vi "map_XY_proc_marmo.vi"() -> ()   [LabVIEW 2011]
panel:
  in  "go to z meas":bool
  in  "find z pos 3":bool
  in  "find z pos 2":bool
  in  "find z pos":bool
  in  "find y pos":bool
  in  "find x pos":bool
  in  "zero y":bool
  in  "zero x":bool
  in  "zero Z":bool
  in  "stop":bool
  out "command":string
  out "output":string
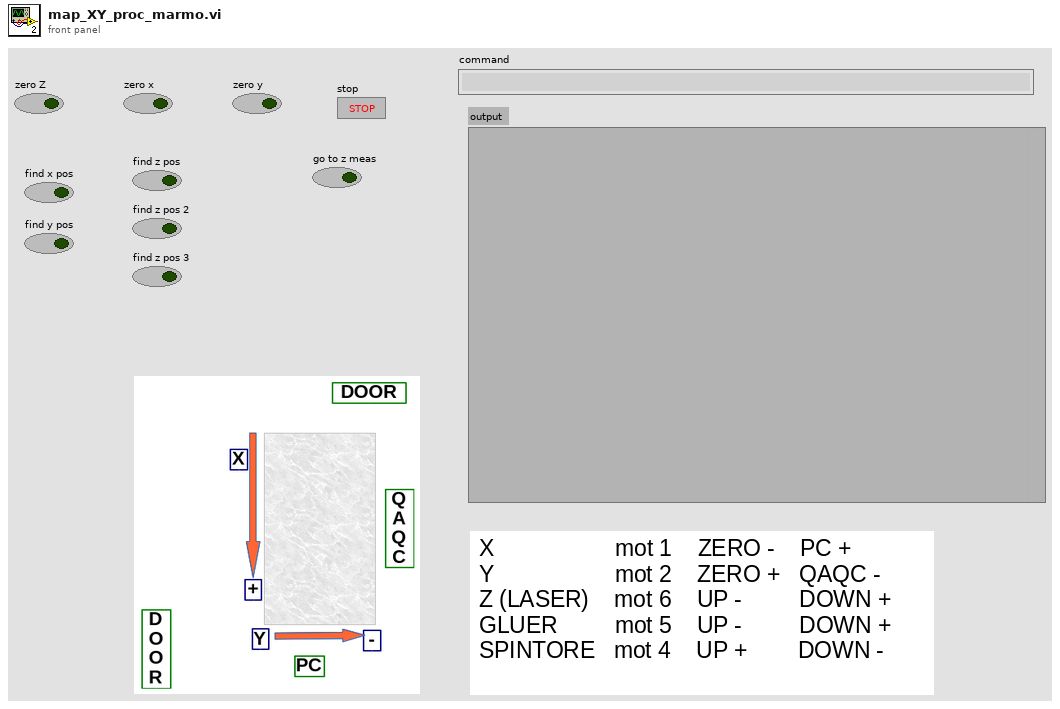
[diagram p1: front panel]
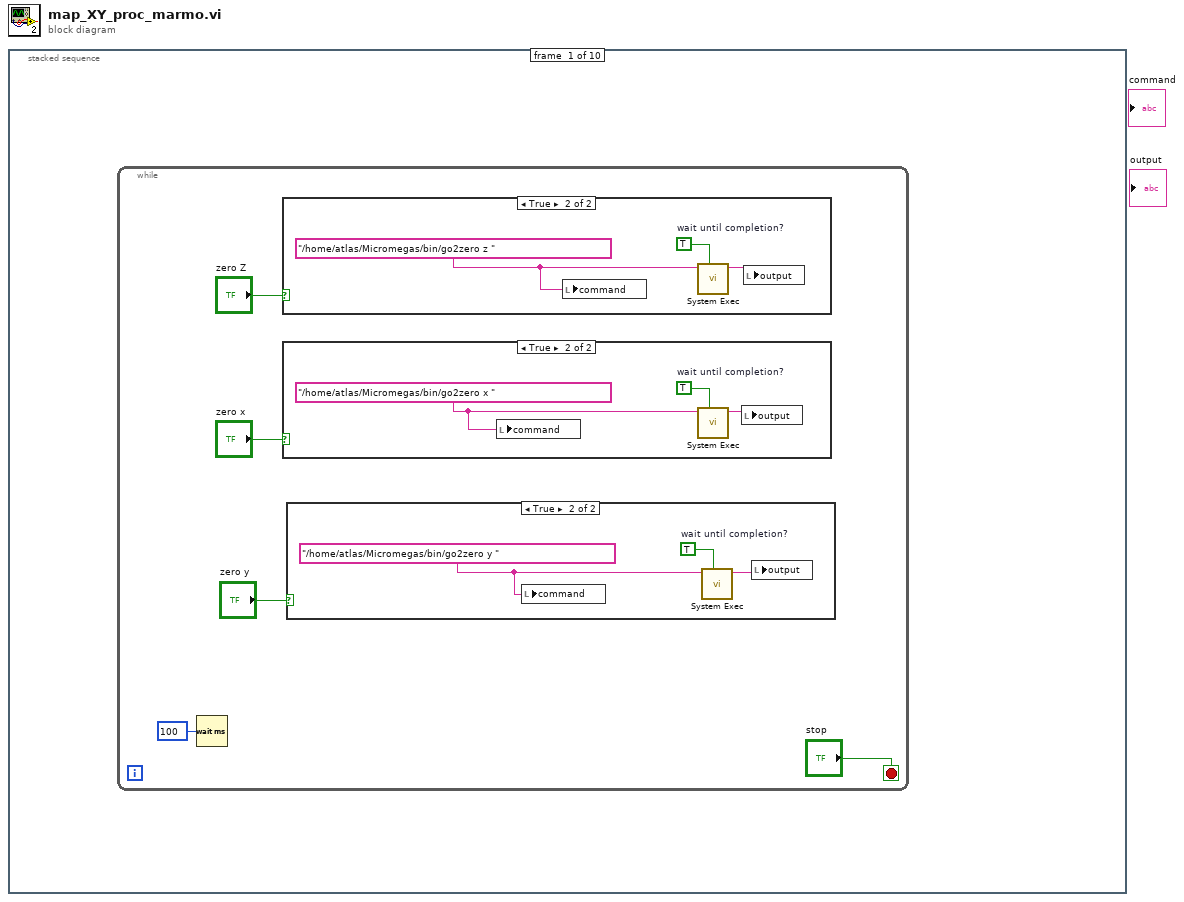
[diagram p0: block diagram]
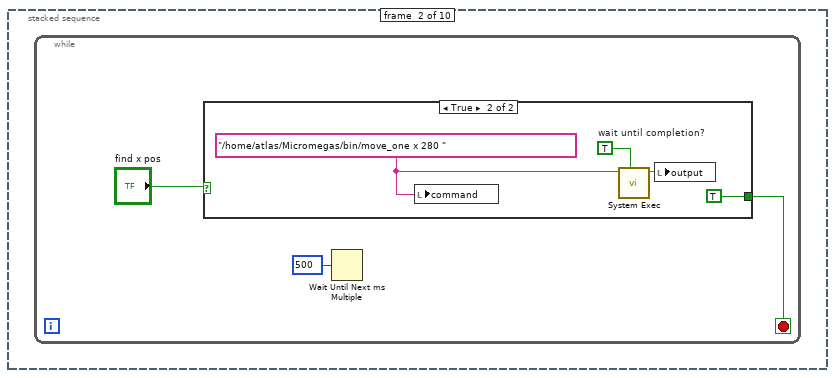
[diagram p5: hidden frame]
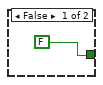
[diagram p6: hidden frame]
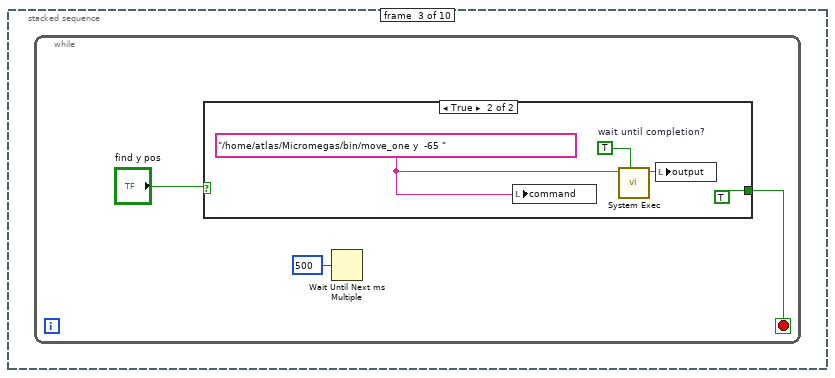
[diagram p7: hidden frame]
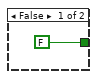
[diagram p8: hidden frame]
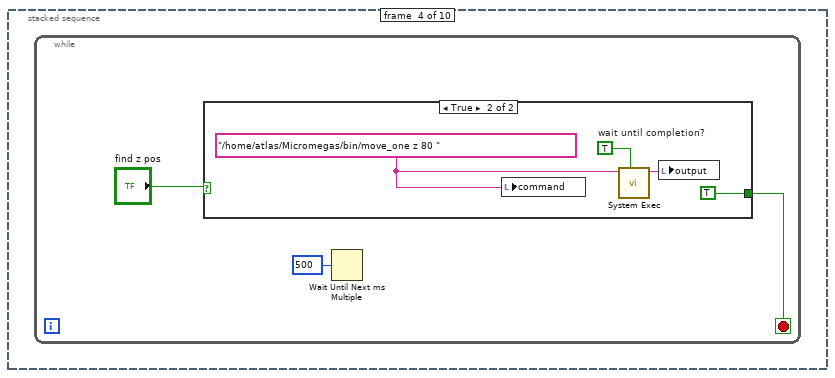
[diagram p9: hidden frame]
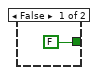
[diagram p10: hidden frame]
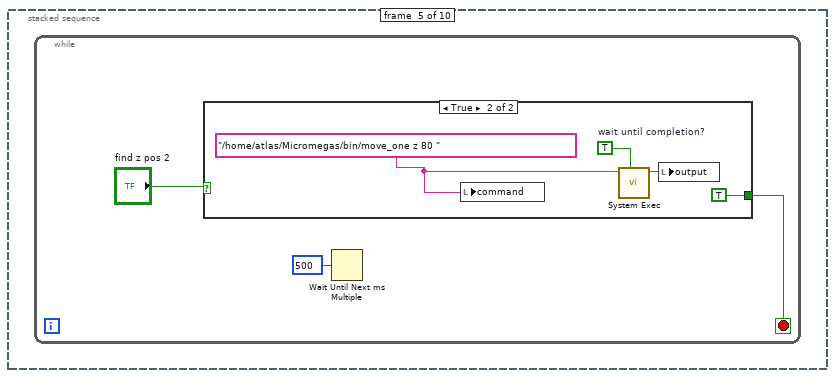
[diagram p11: hidden frame]
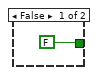
[diagram p12: hidden frame]
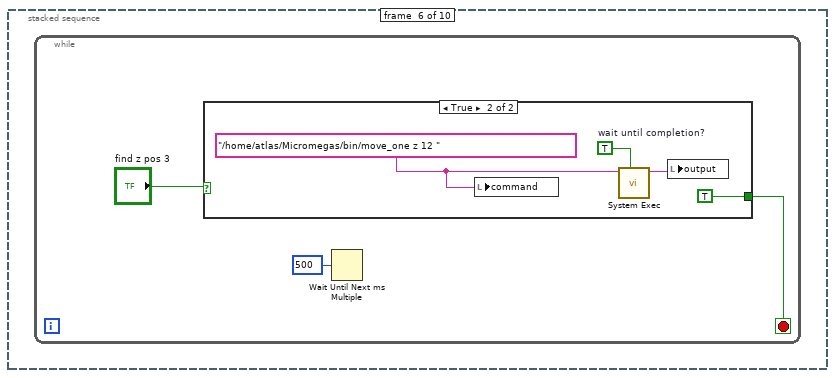
[diagram p13: hidden frame]
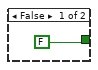
[diagram p14: hidden frame]
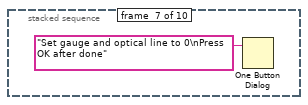
[diagram p15: hidden frame]
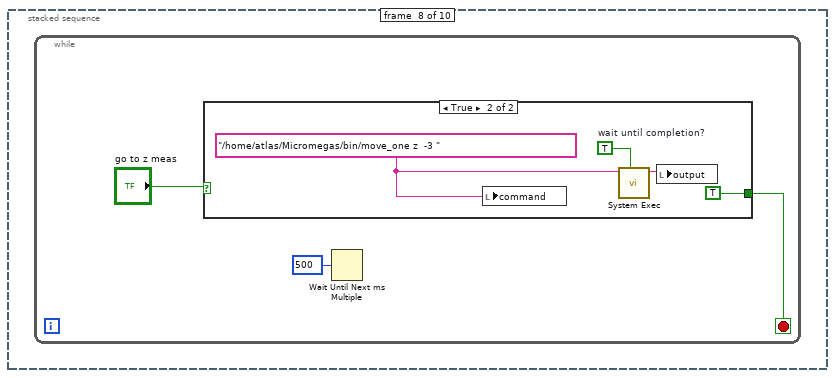
[diagram p16: hidden frame]
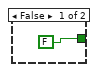
[diagram p17: hidden frame]
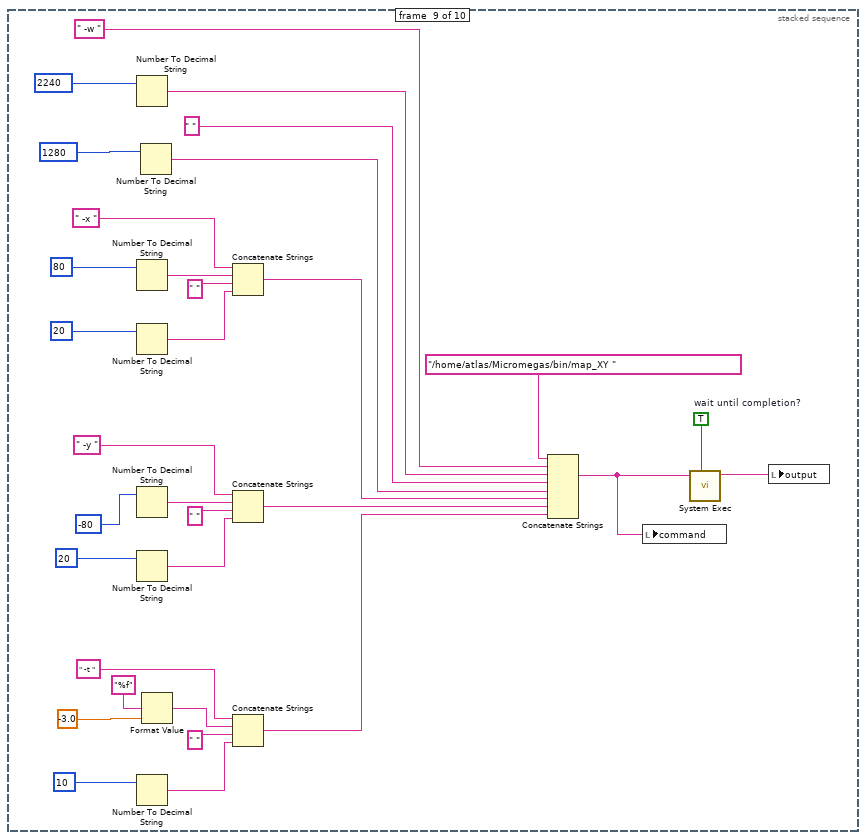
[diagram p18: hidden frame]
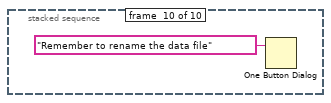
[diagram p19: hidden frame]
diagram:
  n1 = stacked-sequence {
    frame #0 {
      n2 = while {
        stop <- "stop" stop-if-true
        n3 = Wait (ms)(milliseconds to wait=u32 100) -> ()  [unwired: 1 out]
        n4 = case shown="True" "zero Z" {
          frame False {
          }
          frame True {
            w13 = "/home/atlas/Micromegas/bin/go2zero z " ("string")
            w14 = TRUE  # wait until completion?
            n5 = local write "command"(w13) -> ()
            n6 = call <vilib>:"System Exec.vi"("wait until completion? (T)"=w14, "command line"=w13) -> ("standard output"=w12:string)  [unwired: 6 in, 3 out]
            n7 = local write "output"(w12) -> ()
          }
        }
        n8 = case shown="True" "zero x" {
          frame False {
          }
          frame True {
            w10 = "/home/atlas/Micromegas/bin/go2zero x " ("string")
            w11 = TRUE  # wait until completion?
            n9 = local write "command"(w10) -> ()
            n10 = call <vilib>:"System Exec.vi"("wait until completion? (T)"=w11, "command line"=w10) -> ("standard output"=w9:string)  [unwired: 6 in, 3 out]
            n11 = local write "output"(w9) -> ()
          }
        }
        n12 = case shown="True" "zero y" {
          frame False {
          }
          frame True {
            w7 = "/home/atlas/Micromegas/bin/go2zero y " ("string")
            w8 = TRUE  # wait until completion?
            n13 = local write "command"(w7) -> ()
            n14 = call <vilib>:"System Exec.vi"("wait until completion? (T)"=w8, "command line"=w7) -> ("standard output"=w6:string)  [unwired: 6 in, 3 out]
            n15 = local write "output"(w6) -> ()
          }
        }
      }
    }
    frame #1 {
      n16 = while {
        stop <- w15 stop-if-true
        n17 = case shown="True" "find x pos" {
          tunnel: [FALSE TRUE] -> w15
          frame False {
          }
          frame True {
            w20 = "/home/atlas/Micromegas/bin/move_one x 280 " ("string")
            w22 = TRUE  # wait until completion?
            n18 = local write "command"(w20) -> ()
            n19 = call <vilib>:"System Exec.vi"("wait until completion? (T)"=w22, "command line"=w20) -> ("standard output"=w21:string)  [unwired: 6 in, 3 out]
            n20 = local write "output"(w21) -> ()
          }
        }
        n21 = Wait Until Next ms Multiple(millisecond multiple=u32 500) -> ()  [unwired: 1 out]
      }
    }
    frame #2 {
      n22 = while {
        stop <- w23 stop-if-true
        n23 = case shown="True" "find y pos" {
          tunnel: [FALSE TRUE] -> w23
          frame False {
          }
          frame True {
            w28 = "/home/atlas/Micromegas/bin/move_one y  -65 " ("string")
            w30 = TRUE  # wait until completion?
            n24 = local write "command"(w28) -> ()
            n25 = call <vilib>:"System Exec.vi"("wait until completion? (T)"=w30, "command line"=w28) -> ("standard output"=w29:string)  [unwired: 6 in, 3 out]
            n26 = local write "output"(w29) -> ()
          }
        }
        n27 = Wait Until Next ms Multiple(millisecond multiple=u32 500) -> ()  [unwired: 1 out]
      }
    }
    frame #3 {
      n28 = while {
        stop <- w31 stop-if-true
        n29 = case shown="True" "find z pos" {
          tunnel: [FALSE TRUE] -> w31
          frame False {
          }
          frame True {
            w36 = "/home/atlas/Micromegas/bin/move_one z 80 " ("string")
            w38 = TRUE  # wait until completion?
            n30 = local write "command"(w36) -> ()
            n31 = call <vilib>:"System Exec.vi"("wait until completion? (T)"=w38, "command line"=w36) -> ("standard output"=w37:string)  [unwired: 6 in, 3 out]
            n32 = local write "output"(w37) -> ()
          }
        }
        n33 = Wait Until Next ms Multiple(millisecond multiple=u32 500) -> ()  [unwired: 1 out]
      }
    }
    frame #4 {
      n34 = while {
        stop <- w39 stop-if-true
        n35 = case shown="True" "find z pos 2" {
          tunnel: [FALSE TRUE] -> w39
          frame False {
          }
          frame True {
            w45 = "/home/atlas/Micromegas/bin/move_one z 80 " ("string")
            w46 = TRUE  # wait until completion?
            n36 = local write "command"(w45) -> ()
            n37 = call <vilib>:"System Exec.vi"("wait until completion? (T)"=w46, "command line"=w45) -> ("standard output"=w44:string)  [unwired: 6 in, 3 out]
            n38 = local write "output"(w44) -> ()
          }
        }
        n39 = Wait Until Next ms Multiple(millisecond multiple=u32 500) -> ()  [unwired: 1 out]
      }
    }
    frame #5 {
      n40 = while {
        stop <- w47 stop-if-true
        n41 = case shown="True" "find z pos 3" {
          tunnel: [FALSE TRUE] -> w47
          frame False {
          }
          frame True {
            w53 = "/home/atlas/Micromegas/bin/move_one z 12 " ("string")
            w54 = TRUE  # wait until completion?
            n42 = local write "command"(w53) -> ()
            n43 = call <vilib>:"System Exec.vi"("wait until completion? (T)"=w54, "command line"=w53) -> ("standard output"=w52:string)  [unwired: 6 in, 3 out]
            n44 = local write "output"(w52) -> ()
          }
        }
        n45 = Wait Until Next ms Multiple(millisecond multiple=u32 500) -> ()  [unwired: 1 out]
      }
    }
    frame #6 {
      n46 = One Button Dialog(message="Set gauge and optical line to 0\nPress OK after done") -> ()  [unwired: 1 in, 1 out]
    }
    frame #7 {
      n47 = while {
        stop <- w56 stop-if-true
        n48 = case shown="True" "go to z meas" {
          tunnel: [FALSE TRUE] -> w56
          frame False {
          }
          frame True {
            w62 = "/home/atlas/Micromegas/bin/move_one z  -3 " ("string")
            w63 = TRUE  # wait until completion?
            n49 = local write "command"(w62) -> ()
            n50 = call <vilib>:"System Exec.vi"("wait until completion? (T)"=w63, "command line"=w62) -> ("standard output"=w61:string)  [unwired: 6 in, 3 out]
            n51 = local write "output"(w61) -> ()
          }
        }
        n52 = Wait Until Next ms Multiple(millisecond multiple=u32 500) -> ()  [unwired: 1 out]
      }
    }
    frame #8 {
      w95 = TRUE  # wait until completion?
      n53 = Number To Decimal String(number=2240 ("max X (mm)")) -> (decimal integer string=w86:string)  [unwired: 1 in]
      n54 = Number To Decimal String(number=i64 80 ("step (mm) 2")) -> (decimal integer string=w82:string)  [unwired: 1 in]
      n55 = Number To Decimal String(number=i64 20 ("velocità (X)")) -> (decimal integer string=w79:string)  [unwired: 1 in]
      n56 = Number To Decimal String(number=i64 -80 ("step (mm)")) -> (decimal integer string=w77:string)  [unwired: 1 in]
      n57 = Number To Decimal String(number=i64 20 ("velocità (Y)")) -> (decimal integer string=w74:string)  [unwired: 1 in]
      n58 = Number To Decimal String(number=i64 10 ("velocità (S)")) -> (decimal integer string=w69:string)  [unwired: 1 in]
      n59 = Number To Decimal String(number=1280 ("max Y (mm)")) -> (decimal integer string=w87:string)  [unwired: 1 in]
      n60 = Format Value(format string="%f", value (0)=-3.0 ("mm (S)")) -> (output string=w65:string)  [unwired: 1 in]
      n61 = Concatenate Strings(" -x " ("string"), w82, " " ("string"), w79) -> (w93:string)
      n62 = Concatenate Strings(" -y " ("string"), w77, " " ("string"), w74) -> (w92:string)
      n63 = Concatenate Strings(" -t " ("string"), w65, " " ("string"), w69) -> (w91:string)
      n64 = Concatenate Strings("/home/atlas/Micromegas/bin/map_XY " ("string"), " -w ", w86, " " ("string"), w87, w93, w92, w91) -> (w84:string)
      n65 = local write "command"(w84) -> ()
      n66 = call <vilib>:"System Exec.vi"("wait until completion? (T)"=w95, "command line"=w84) -> ("standard output"=w64:string)  [unwired: 6 in, 3 out]
      n67 = local write "output"(w64) -> ()
    }
    frame #9 {
      n68 = One Button Dialog(message="Remember to rename the data file") -> ()  [unwired: 1 in, 1 out]
    }
  }
